vi "Get UI Control Value.vi"(8 "error in (no error)":errorcluster, 10 "VI Ref":refnum<vi>, 11 "Double Parameter in":refnum<class "Double Array Parameter.lvclass">) -> (0 "error out":errorcluster, 3 "Double Parameter out":refnum<class "Double Array Parameter.lvclass">)   [LabVIEW 2019, in "CD Parameter Manager API.lvlib" / "Double Array Parameter.lvclass"]
uses:
  Double Array Parameter.lvclass
  C:/Repositories/UI-Control-Initializer-API/Source/Parameter Class/Parameter.lvclass
  Parameter Class/Parameter.lvclass/Parameter.ctl
  Double Array Parameter.lvclass/Double Array Parameter.ctl
  Parameter Class/Member Accessors/Read Control label.vi
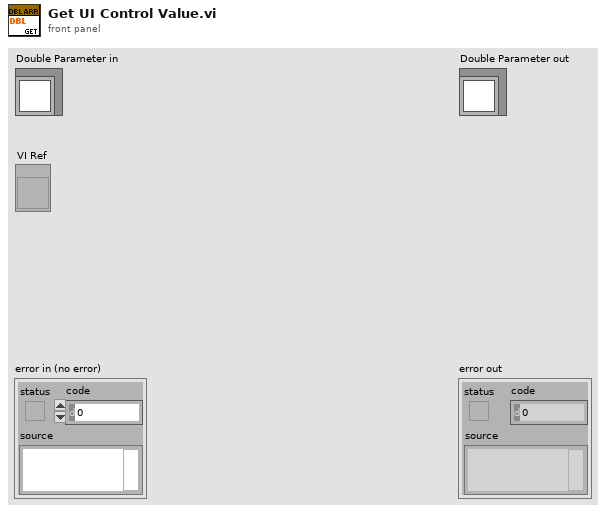
[diagram p1: front panel]
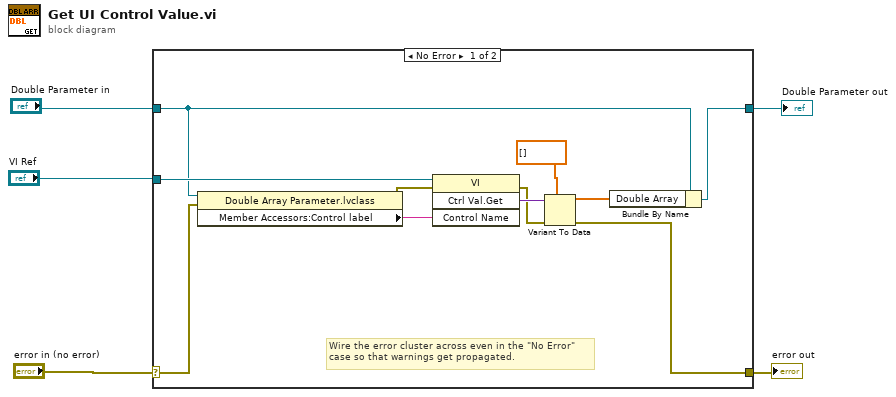
[diagram p0: block diagram]
diagram:
  n1 = case shown="No Error" "error in (no error)" {
    selector: "error in (no error)" -> [w10 w18]
    tunnel: [w7 w18] -> w5
    tunnel: [w15 w17] -> w4
    tunnel: "Double Parameter in" -> [w9 w17]
    tunnel: "VI Ref" -> [w16 _]
    frame No Error {
      # "Wire the error cluster across even in the \"No Error\"\ncase so that warnings get propagated."
      n2 = property class="Double Array Parameter.lvclass"(reference=w9, error in=w10) -> (error out=w11:errorcluster, "Member Accessors:Control label"=w12:string)  [unwired: 1 out]
      n3 = invoke class="VI" method="Ctrl Val.Get"(reference=w16, error in=w11, "Control Name"=w12) -> (error out=w8:errorcluster, "Get Control Value Variant"=w14:variant)  [unwired: 1 in, 2 out]
      n4 = Variant To Data(error in=w8, type=dbl[] [], Variant=w14) -> (data=w13:dbl[], error out=w7:errorcluster)
      n5 = Bundle By Name(cluster=w9, "Double Array"=w13) -> (w15:refnum<class "Double Array Parameter.lvclass">)
    }
    frame Error {
    }
  }
  "error out" <- w5
  "Double Parameter out" <- w4
